vi "Add Modules.vi"(8 "error in (no error)":errorcluster, 10 "Refs":T1, 11 "IO Loop in":refnum<class "Module Loop.lvclass">) -> (0 "error out":errorcluster, 2 "Mod.Locals.Ref":refnum<vi>[](array[refnum]), 3 "IO Loop out":refnum<class "Module Loop.lvclass">)   [LabVIEW 2015, in "Module Loop.lvclass"]
uses:
  Module Loop.lvclass
  VI/BlockDiagram.Refs.ctl
  VI/Module.Refs.ctl
  <vilib>/Utility/miscctls.llb/LVPointTypeDef.ctl
  Read Modules.vi
  Module/Module/Module.lvclass
  VI/VI.lvclass
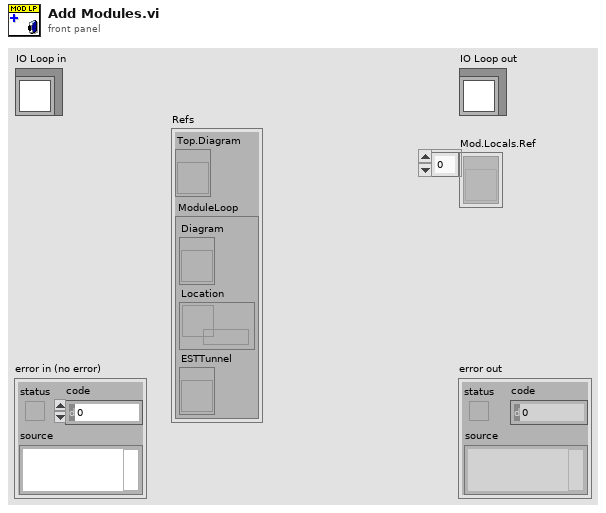
[diagram p1: front panel]
types:
  T1 = typedef "VI.lvclass/BlockDiagram.Refs.ctl" = cluster{"Top.Diagram":refnum<vi>, "ModuleLoop":T2}
  T2 = typedef "VI.lvclass/Module.Refs.ctl" = cluster{"Diagram":refnum<vi>, "Location":refnum<data-value>, "ESTTunnel":refnum<vi>}
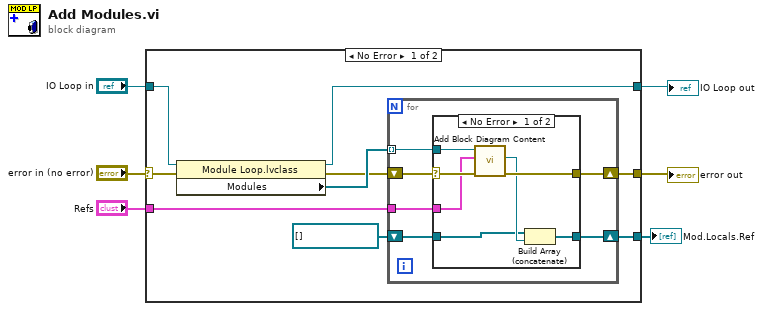
[diagram p0: block diagram]
diagram:
  n1 = case shown="No Error" "error in (no error)" {
    selector: "error in (no error)" -> [w13 w32]
    tunnel: [w12 w32] -> w5
    tunnel: [w10 w31] -> w3
    tunnel: "IO Loop in" -> [w14 w31]
    tunnel: "Refs" -> [w9 _]
    tunnel: [w7 _] -> w1
    frame No Error {
      n2 = property class="Module Loop.lvclass"(reference=w14, error in=w13) -> (reference out=w10:refnum<class "Module Loop.lvclass">, error out=w11:errorcluster, "Modules"=w15:refnum<class "Module.lvclass">[])
      n3 = for {
        tunnel: w15 -> [w20] mode=indexing
        shift-right: [w19] -> w12
        shift-left: w11 -> [w21]
        tunnel: w9 -> [w18]
        shift-right: [w17] -> w7
        shift-left: refnum<vi>[] [] -> [w16]
        n4 = case shown="No Error" w21 {
          selector: w21 -> [w28 w30]
          tunnel: [w26 w30] -> w19
          tunnel: w20 -> [w27 _]
          tunnel: w18 -> [w25 _]
          tunnel: [w23 w29] -> w17
          tunnel: w16 -> [w22 w29]
          frame No Error {
            n5 = call-dynamic "Add Block Diagram Content.vi"("error in (no error)"=w28, "Refs"=w25, "Module in"=w27) -> ("error out"=w26:errorcluster, "Local.Ref"=w24:refnum<vi>)  [unwired: 6 in, 1 out]
            n6 = Build Array (concatenate)(w22, w24) -> (w23:refnum<vi>[])
          }
          frame Error {
          }
        }
      }
    }
    frame Error {
    }
  }
  "error out" <- w5
  "IO Loop out" <- w3
  "Mod.Locals.Ref" <- w1
